vi "Benchmark - Delta Time.vi"() -> ()   [LabVIEW 2020, in "Utility.lvlib"]
uses:
  Utility.lvlib
  <vilib>/Analysis/NI_AALBase.lvlib
  8ca8b4a3-a15b-4534-87bf-3f66f767895e.vi
panel:
  out "Std Dev":dbl format="%.1p"
  out "Mean":dbl format="%.1p"
  out "Histogram Graph":T1(graph)
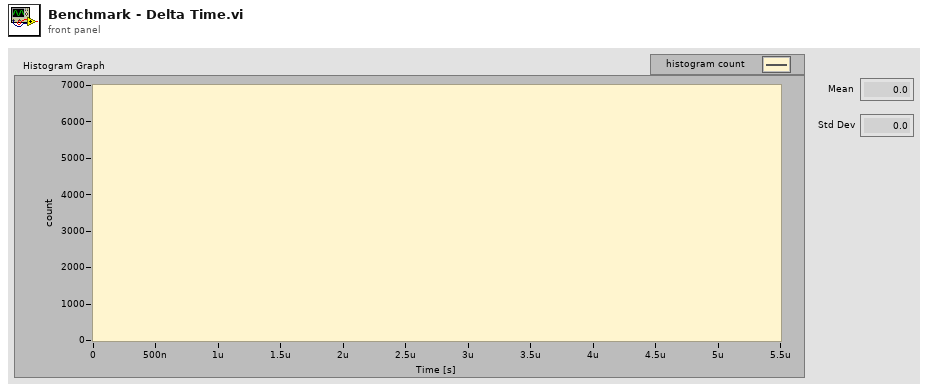
[diagram p1: front panel]
types:
  T1 = cluster{"X Values":dbl[], "Histogram: h(x)":i32[]}
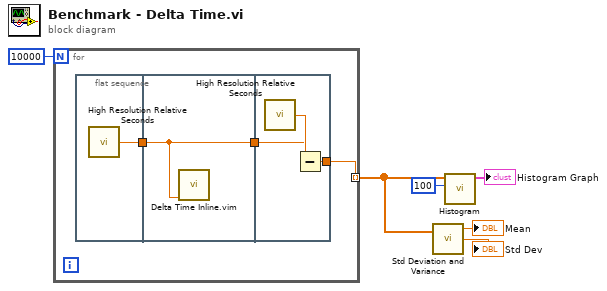
[diagram p0: block diagram]
diagram:
  n1 = for {
    N: 10000 -> [_]
    tunnel: [w7] -> w3 mode=indexing
    n2 = flat-sequence {
      tunnel: [w10] -> w9
      tunnel: w9 -> [w11]
      tunnel: [w11] -> w8
      tunnel: w8 -> [w13]
      tunnel: [w12] -> w7
      frame #0 {
        n3 = call <vilib>:"High Resolution Relative Seconds.vi"() -> ("relative seconds"=w10:dbl)
      }
      frame #1 {
        n4 = call "Delta Time Inline.vim"("value in"=w11) -> ()  [unwired: 8 in, 3 out]
      }
      frame #2 {
        n5 = call <vilib>:"High Resolution Relative Seconds.vi"() -> ("relative seconds"=w14:dbl)
        n6 = Subtract(x=w14, y=w13) -> (x-y=w12:dbl)
      }
    }
  }
  n7 = call <vilib>:"Std Deviation and Variance.vi"("X"=w3) -> ("mean"=→"Mean":dbl, "standard deviation"=→"Std Dev":dbl)  [unwired: 1 in, 1 out]
  n8 = call <vilib>:"Histogram.vi"("intervals"=100, "X"=w3) -> ("Histogram Graph"=→"Histogram Graph":T1)  [unwired: 6 in, 3 out]
